vi "Edit-dialog.vi"(8 "error in (no error)":errorcluster, 11 "Action in":refnum<class "Move-Timer.lvclass">) -> (0 "error out":errorcluster, 3 "Action out":refnum<class "Move-Timer.lvclass">)   [LabVIEW 2013, in "PowderDeposition.lvlib" / "Move-Timer.lvclass"]
uses:
  Move-Timer.lvclass
  Move-Timer-settings.ctl
  Move-Timer.lvclass/Move-Timer.ctl
panel:
  in  "Cancel":bool
  in  "OK":bool
  in  "Edit dialog":T1
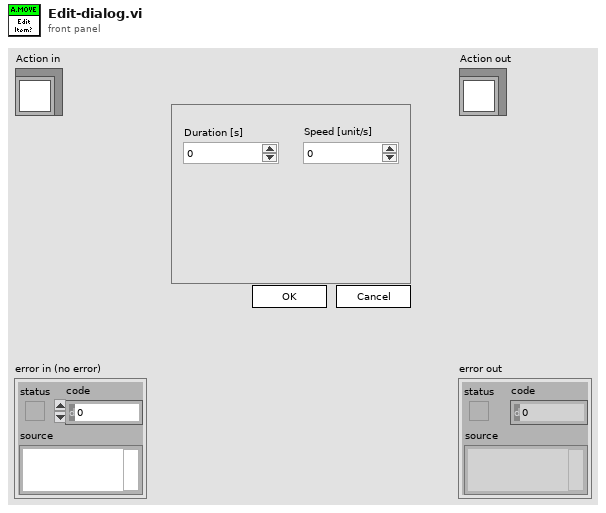
[diagram p1: front panel]
types:
  T1 = typedef "PowderDeposition.lvlib/Move-Timer.lvclass/Move-Timer-settings.ctl" = cluster{"Duration [s]":dbl, "Speed":dbl}
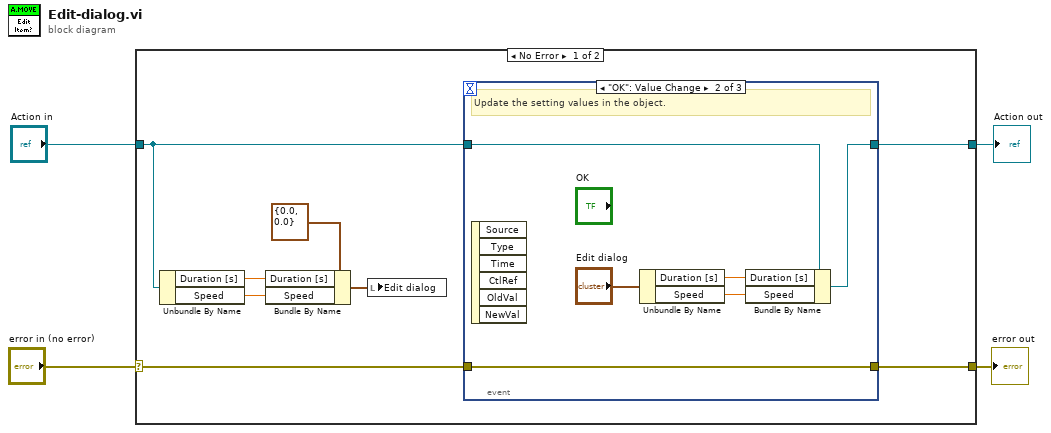
[diagram p0: block diagram]
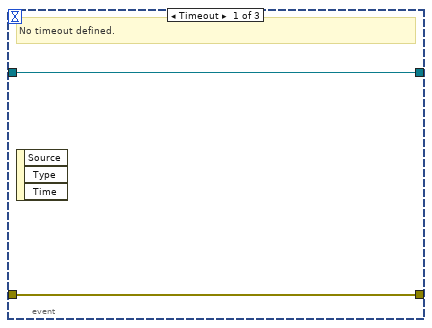
[diagram p2: hidden frame]
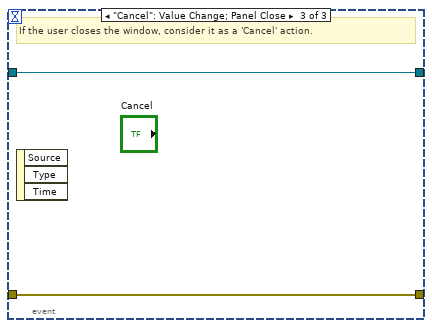
[diagram p3: hidden frame]
diagram:
  n1 = case shown="No Error" "error in (no error)" {
    selector: "error in (no error)" -> [w11 w24]
    tunnel: [w10 w24] -> w3
    tunnel: [w12 w23] -> w1
    tunnel: "Action in" -> [w7 w23]
    frame No Error {
      n2 = Unbundle By Name(w7) -> ("Duration [s]"=w8:dbl, "Speed"=w9:dbl)
      n3 = Bundle By Name(cluster=T1 {"Duration [s]"=0.0, "Speed"=0.0} ("Edit dialog"), "Duration [s]"=w8, "Speed"=w9) -> (w5:T1)
      n4 = local write "Edit dialog"(w5) -> ()
      n5 = event shown="[1] \"OK\": Value Change" {
        selector: _ -> [_ _ _]
        dyn-events: _ -> [_ _ _]
        timeout: _ -> [_ _ _]
        tunnel: w7 -> [w14 w19 w22]
        tunnel: [w14 w18 w22] -> w12
        tunnel: w11 -> [w13 w20 w21]
        tunnel: [w13 w20 w21] -> w10
        event Timeout {
          # "No timeout defined."
          n6 = event-data() -> ()  [unwired: 1 in, 3 out]
        }
        event "OK": Value Change {
          # "Update the setting values in the object."
          n7 = event-data() -> ()  [unwired: 1 in, 6 out]
          n8 = Unbundle By Name("Edit dialog") -> ("Duration [s]"=w16:dbl, "Speed"=w15:dbl)
          n9 = Bundle By Name(cluster=w19, "Duration [s]"=w16, "Speed"=w15) -> (w18:refnum<class "Move-Timer.lvclass">)
        }
        event "Cancel": Value Change; Panel Close {
          # "If the user closes the window, consider it as a 'Cancel' action."
          n10 = event-data() -> ()  [unwired: 1 in, 3 out]
        }
      }
    }
    frame Error {
    }
  }
  "error out" <- w3
  "Action out" <- w1
